vi "Linear Regression for Load Cell.vi"(8 "x3":dbl[](array[numeric]), 9 "x2":dbl[](array[numeric]), 10 "X1":dbl[](array[numeric]), 11 "slope-intercept":dbl[][](array[numeric])) -> (1 "Force HL":dbl[](array[numeric]), 2 "Force HR":dbl[](array[numeric]), 3 "Force Forepaw":dbl[](array[numeric]))   [LabVIEW 2015]
uses:
  <vilib>/express/express arith-compare/Formula/XNode/ExpressFormulaBlockNode.xnode
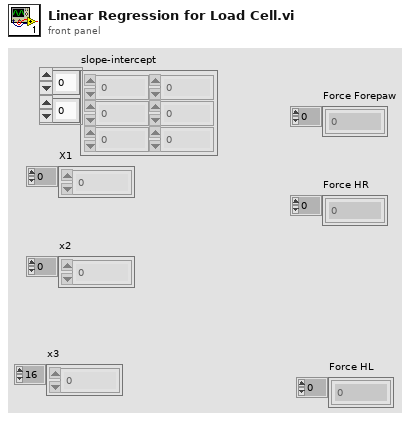
[diagram p1: front panel]
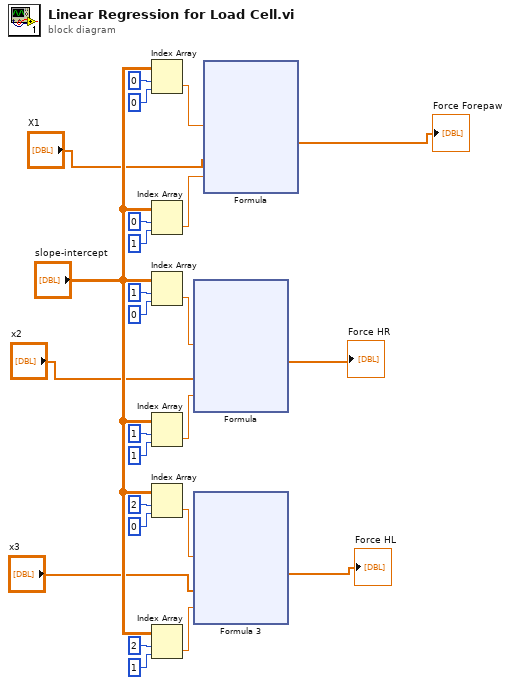
[diagram p0: block diagram]
diagram:
  n1 = Index Array(array="slope-intercept", index (row)=0, index (col)=0) -> (element=w11:dbl)
  n2 = Index Array(array="slope-intercept", index (row)=0, index (col)=1 ("disabled index (col)")) -> (element=w12:dbl)
  n3 = Index Array(array="slope-intercept", index (row)=1, index (col)=0 ("disabled index (col)")) -> (element=w9:dbl)
  n4 = Index Array(array="slope-intercept", index (row)=1, index (col)=1 ("disabled index (col)")) -> (element=w10:dbl)
  n5 = Index Array(array="slope-intercept", index (row)=2, index (col)=0) -> (element=w7:dbl)
  n6 = Index Array(array="slope-intercept", index (row)=2, index (col)=1) -> (element=w8:dbl)
  n7 = xnode "Formula"("m2"=w9, "x2"="x2", "b2"=w10) -> ("Result"=→"Force HR":dbl[])  [unwired: 1 in, 1 out]
  n8 = xnode "Formula 3"("m3"=w7, "x3"="x3", "b3"=w8) -> ("Result"=→"Force HL":dbl[])  [unwired: 1 in, 1 out]
  n9 = xnode "Formula"("m1"=w11, "x1"="X1", "b1"=w12) -> ("Result"=→"Force Forepaw":dbl[])  [unwired: 1 in, 1 out]
